vi "HEAD.vi"(6 "timeout (10000)":i32=10000, 8 "error in (no error)":errorcluster, 10 "url":string, 11 "HTTP Client Abstract in":refnum<class "Abstract HTTP Client.lvclass">) -> (0 "error out":errorcluster, 2 "headers":string, 3 "HTTP Client Abstract out":refnum<class "Abstract HTTP Client.lvclass">, 4 "status code":u32)   [LabVIEW 2020, in "HTTP Client Abstract.lvlib" / "Abstract HTTP Client.lvclass"]
uses:
  Abstract HTTP Client.lvclass
  Abstract HTTP Client.lvclass/Abstract HTTP Client.ctl
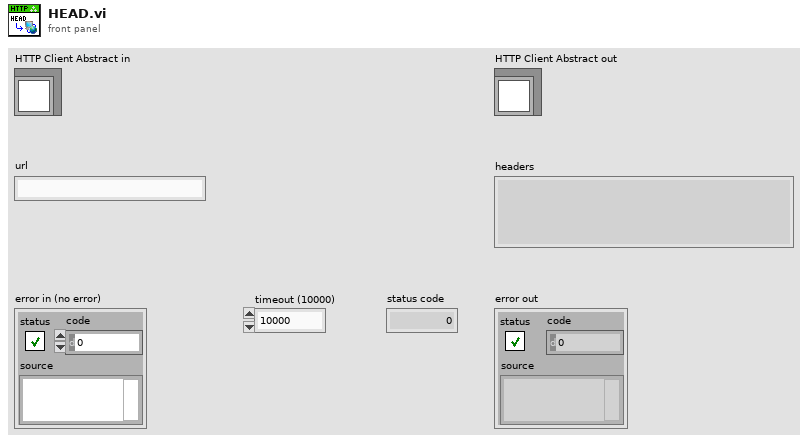
[diagram p1: front panel]
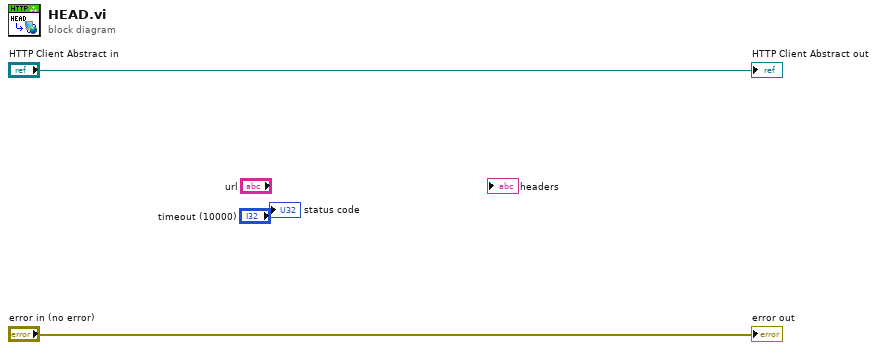
[diagram p0: block diagram]
diagram:
  "error out" <- "error in (no error)"
  "HTTP Client Abstract out" <- "HTTP Client Abstract in"
